vi "getYScaleRange.vi"(8 "error in (no error)":errorcluster, 11 "QControl_Graph in":refnum<class "QControl_Graph.lvclass">) -> (0 "error out":errorcluster, 2 "YScale Range":cluster{"Maximum":dbl, "Minimum":dbl}, 3 "QControl_Graph out":refnum<class "QControl_Graph.lvclass">)   [LabVIEW 2017, in "QControl_Graph.lvclass"]
uses:
  QControl_Graph.lvclass
  C:/Program Files (x86)/National Instruments/LabVIEW 2017/vi.lib/QSI/QControls/QControl Classes/GraphChart/GraphChart.lvclass
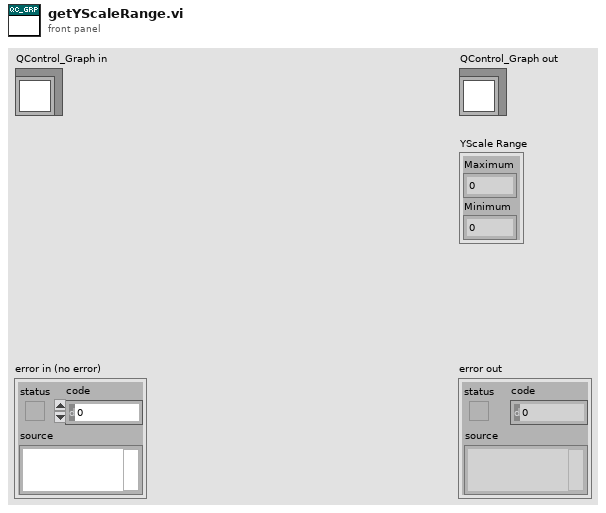
[diagram p1: front panel]
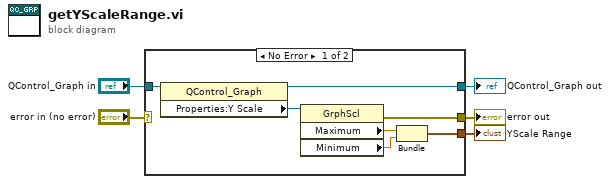
[diagram p0: block diagram]
diagram:
  n1 = case shown="No Error" "error in (no error)" {
    selector: "error in (no error)" -> [_ w14]
    tunnel: [w6 w14] -> w4
    tunnel: [w11 w13] -> w2
    tunnel: "QControl_Graph in" -> [w12 w13]
    tunnel: [w7 _] -> w1
    frame No Error {
      n2 = property on="Property Node" class="QControl_Graph"(reference=w12) -> (reference out=w11:refnum<class "QControl_Graph.lvclass">, "Properties:Y Scale"=w10:refnum<vi>)  [unwired: 1 in, 1 out]
      n3 = property class="GrphScl"(reference=w10) -> (error out=w6:errorcluster, "Maximum"=w9:dbl, "Minimum"=w8:dbl)  [unwired: 1 in, 1 out]
      n4 = Bundle("Maximum"=w9, "Minimum"=w8) -> (w7:cluster{"Maximum":dbl, "Minimum":dbl})  [unwired: 1 in]
    }
    frame Error {
    }
  }
  "error out" <- w4
  "QControl_Graph out" <- w2
  "YScale Range" <- w1
